vi "connect.vi"(5 "module path":path, 7 "Python version":string, 8 "error in (no error)":errorcluster, 9 "password":string="abracadabra", 10 "port":i32=50000, 11 "ip_address":string="localhost") -> (0 "error out":errorcluster, 3 "py out":T1)   [LabVIEW 2022 SP3, in "pythonq.lvlib"]
uses:
  pythonq.lvlib
  py_session.ctl
  py_cluster.ctl
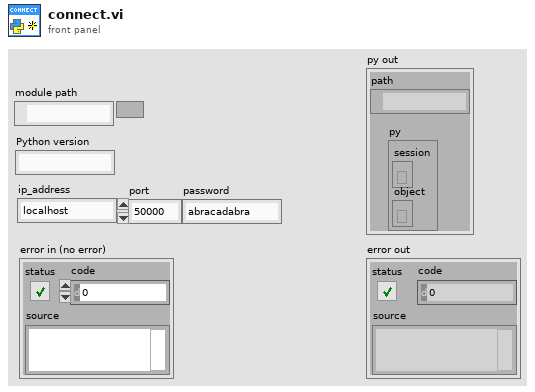
[diagram p1: front panel]
types:
  T1 = typedef "pythonq.lvlib/py_cluster.ctl" = cluster{"path":path, "py":T2}
  T2 = typedef "pythonq.lvlib/py_session.ctl" = cluster{"session":refnum<k35>, "object":refnum<k38>}
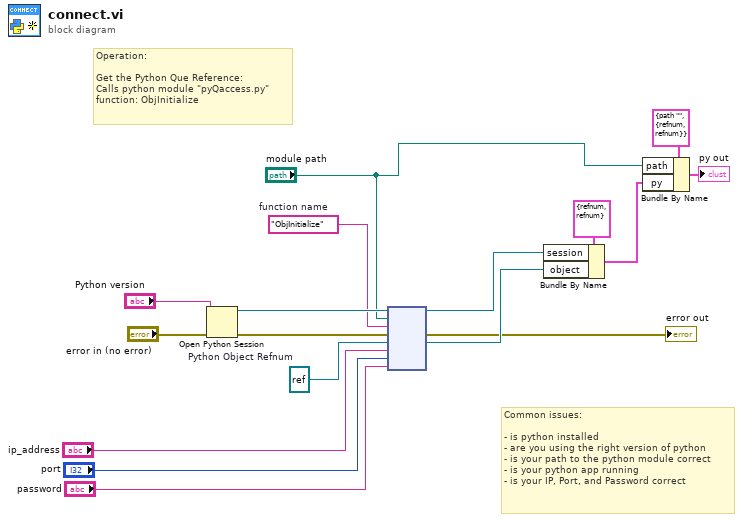
[diagram p0: block diagram]
diagram:
  w13 = refnum<k38> refnum  # Python Object Refnum
  w14 = "ObjInitialize"  # function name
  # "Common issues:\n\n- is python installed\n- are you using the right version of python\n- is your path to the python module correct\n- is your python app running\n- is your IP, Port, and Password correct"
  # "Operation:\n\nGet the Python Que Reference:\nCalls python module \"pyQaccess.py\"\nfunction: ObjInitialize"
  n1 = Open Python Session(python version="Python version", 3:"error in (no error)") -> (session out=w16:refnum<k35>, error out=w15:errorcluster)  [unwired: 1 in]
  n2 = node(w16, "module path", w14, w15, w13, "ip_address", "port", "password") -> (w8:refnum<k35>, →"error out":errorcluster, w7:refnum<k38>)  [unwired: 3 in, 2 out]
  n3 = Bundle By Name(cluster=T2 {"session"=refnum, "object"=refnum} ("Cluster"), "session"=w8, "object"=w7) -> (w3:T2)
  n4 = Bundle By Name(cluster=T1 {"path"=path "", "py"={"session"=refnum, "object"=refnum}} ("Cluster"), "path"="module path", "py"=w3) -> (→"py out":T1)
